vi "rest_get_devices.vi"(8 "error in":errorcluster, 11 "Base URL":string="http://localhost:5001/") -> (0 "error out":errorcluster, 2 "DeviceArray":string[](array[string]))   [LabVIEW 2024]
uses:
  <vilib>/addons/_JKI.lib/REST Client/classes/REST Client/REST Client.lvclass
panel:
  out "Menu Ring":u16(ring) items=["esp32-abcd01", "esp32-abcd03", "esp32-abcd02"]
  out "Devices":cluster{"device_id":string}[](array[cluster])
  out "Response body":string
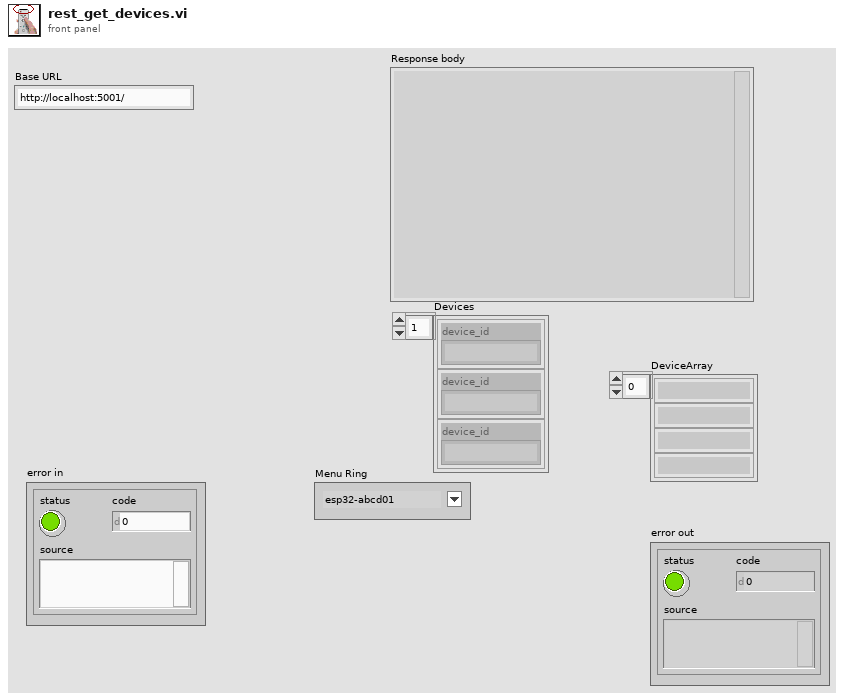
[diagram p1: front panel]
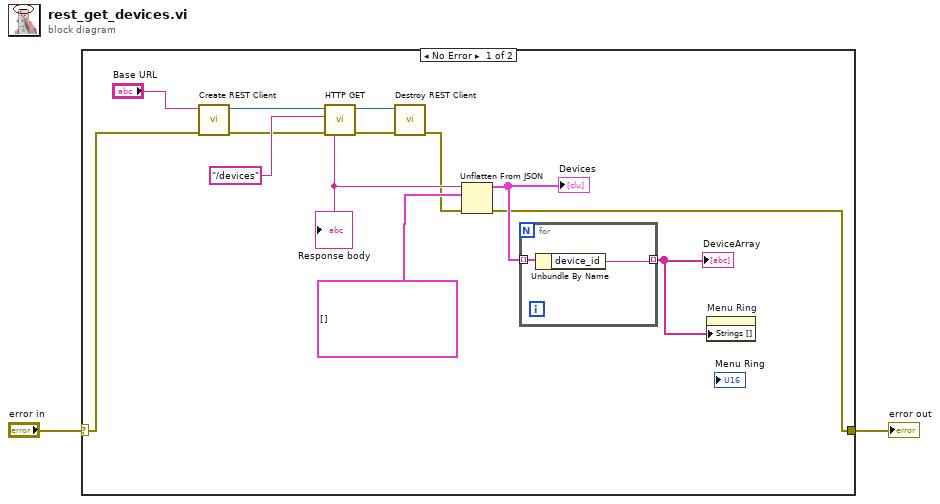
[diagram p0: block diagram]
diagram:
  n1 = case shown="No Error" "error in" {
    selector: "error in" -> [w7 w18]
    tunnel: [w3 w18] -> w1
    frame No Error {
      n2 = call <vilib>:"Create REST Client.vi"("error in (no error)"=w7, "Base URL"="Base URL") -> ("error out"=w6:errorcluster, "REST Client out"=w15:refnum<class "REST Client.lvclass">)  [unwired: 8 in]
      n3 = call-dynamic "HTTP GET.vi"("error in (no error)"=w6, "Path"="/devices", "REST Client in"=w15) -> ("error out"=w5:errorcluster, "Response body"=w11:string, "REST Client out"=w14:refnum<class "REST Client.lvclass">)  [unwired: 3 in, 3 out]
      "Response body" <- w11
      n4 = call-dynamic "Destroy REST Client.vi"("error in (no error)"=w5, "REST Client in"=w14) -> ("error out"=w4:errorcluster)  [unwired: 9 in]
      n5 = Unflatten From JSON(JSON string=w11, type and defaults=cluster{"device_id":string}[] [], error in (no error)=w4) -> (value=w9:cluster{"device_id":string}[], error out=w3:errorcluster)  [unwired: 4 in]
      "Devices" <- w9
      n6 = for {
        tunnel: w9 -> [w17] mode=indexing
        tunnel: [w16] -> w8 mode=indexing
        n7 = Unbundle By Name(w17) -> ("device_id"=w16:string)
      }
      "DeviceArray" <- w8
      n8 = property on="Menu Ring" class="Ring (strict)"("Strings []"=w8) -> ()  [unwired: 2 in, 2 out]
    }
    frame Error {
    }
  }
  "error out" <- w1
